vi "Close.vi"(8 "error in":errorcluster, 11 "Power Setpoint in":refnum<class "Power Setpoint.lvclass">) -> (0 "error out":errorcluster, 3 "Power Setpoint out":refnum<class "Power Setpoint.lvclass">)   [LabVIEW 2023, in "Power Setpoint.lvclass"]
uses:
  Power Setpoint.lvclass
  Parents/Setpoint/Setpoint.lvclass
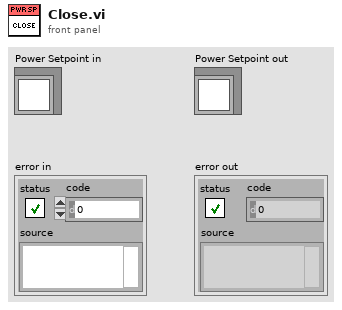
[diagram p1: front panel]
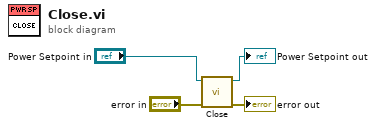
[diagram p0: block diagram]
diagram:
  n1 = call-parent "Close.vi"("error in"="error in", "Setpoint in"="Power Setpoint in") -> ("error out"=→"error out":errorcluster, "Setpoint out"=→"Power Setpoint out":refnum<class "Power Setpoint.lvclass">)  [unwired: 8 in]
